vi "SlicePlane.vi"(0 "Plane dimensions (cm)":cluster{"x":dbl, "y":dbl, "z":dbl}={"x"=0.2, "y"=0.0, "z"=0.2} {"x" format="%.2f"; "z" format="%.2f"; "y" format="%.2f"}, 1 "strip (cm)":cluster{"radius":dbl, "h":dbl, "a":dbl}={"radius"=9.0, "h"=2.0, "a"=4.0} {"radius" format="%.2f"; "a" format="%.4f"; "h" format="%.4f"}, 2 "Plane":u16(ring)=2 items=["X-Y", "Z-Y", "X-Z"], 3 "freq (MHz)":dbl=4.7 format="%.2f", 4 "Geometry":u16(ring)=1 items=["single wedge", "dual wedge", "Outer Rec Hole", "Inner Rect Hole", "single strip", "dual strips", "Cap w/ Rect Cut", "middle pair", "middle w/ circ hole"], 6 "Points \t1":i32=10, 7 "Variables":T1={"sound spd (cm/s)"=150000, "time step (s)"=1e-09} {"time step (s)" format="%.2e"}, 8 "Points 2":i32=10, 14 "3D Surface":refnum<k7>(container)) -> (19 "raw data":dbl[][](array[numeric]) format="%.2f")   [LabVIEW 2022 SP3]
uses:
  <vilib>/Analysis/2dsp.llb/1D Convolution (DBL).vi
  <vilib>/Utility/file.llb/Write To Spreadsheet File (DBL).vi
  <vilib>/Platform/NI_3dgraph.lvlib
  <vilib>/Analysis/NI_AALBase.lvlib
  <vilib>/Analysis/NI_AALPro.lvlib
panel:
  in  "Case Constant\n(See Context Help)":bool
  in  "Boolean":bool
  out "data with axis":dbl[][](array[numeric]) format="%.4f"
  in  "save image":bool
  out "axial width (cm)":dbl format="%.4f"
  in  "lower h of strip or outer a":dbl format="%.2f"
  in  "Save Sheet":bool
  out "axial peak (cm)":dbl format="%.2f"
  out "3 dB beamwidth (cm)":dbl format="%.4f"
  out "lateral pressure (y or y or z)":cluster{"output":dbl[], "output":dbl[]}(graph)
  out "axial pressure (x or z or x)":cluster{dbl[], "output":dbl[]}(graph)
  # "y\ny\nz"
  # "x\nz\nx"
  # "For X-Y Pts 1 is for X and Pts 2 is for Y etc."
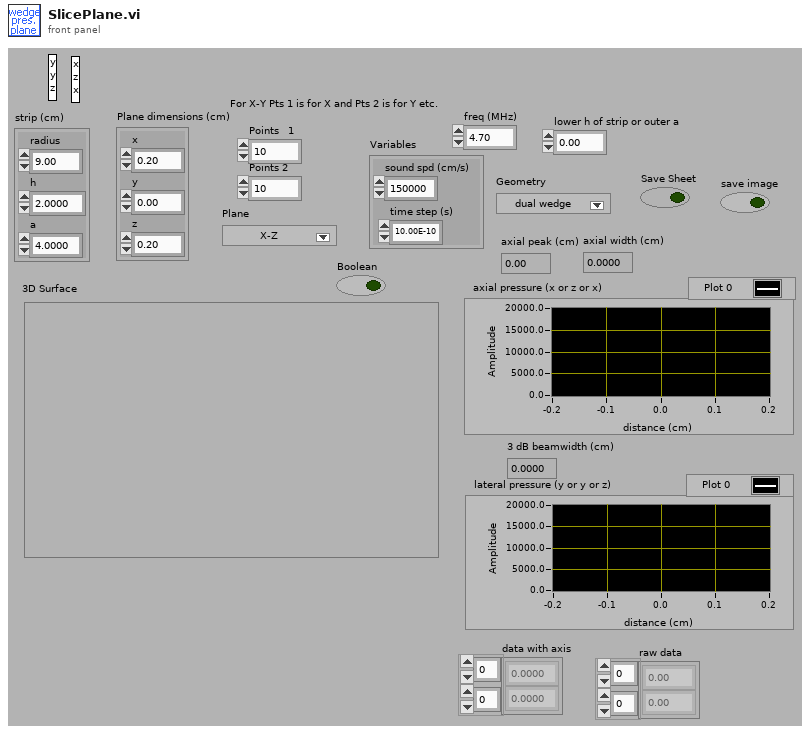
[diagram p1: front panel]
types:
  T1 = cluster{"sound spd (cm/s)":i32, "time step (s)":sgl}
  T2 = cluster{"Number of rings":i32, "sound spd (cm/s)":i32, "z span (cm)":dbl, "z steps":i32, "y span (cm)":dbl, "y steps":i32, "time step (s)":sgl, "z":dbl, "y":dbl, "ref delay":dbl, "freq (MHz)":dbl, "cycles":i32}
  T3 = cluster{"fixed plane":dbl, "fixed plane":dbl, "fixed plane":dbl}
  T4 = cluster{"axial pressure (z)":cluster{dbl[], "output":dbl[]}, "3 dB beamwidth (cm)":dbl, "lateral pressure (y)":cluster{"output":dbl[], "output":dbl[]}, "3 dB beamwidth (cm)":dbl}
  T5 = enum32{"existing file", "new file", "new or existing file", "existing dir", "new dir", "new or existing dir", "existing file (use LLBs)", "new file (use LLBs)", "new or existing file (use LLBs)", "new or existing file or directory (use LLBs)"}
  T6 = typedef "LVRectTypeDef.ctl" = cluster{"left":i16, "top":i16, "right":i16, "bottom":i16}
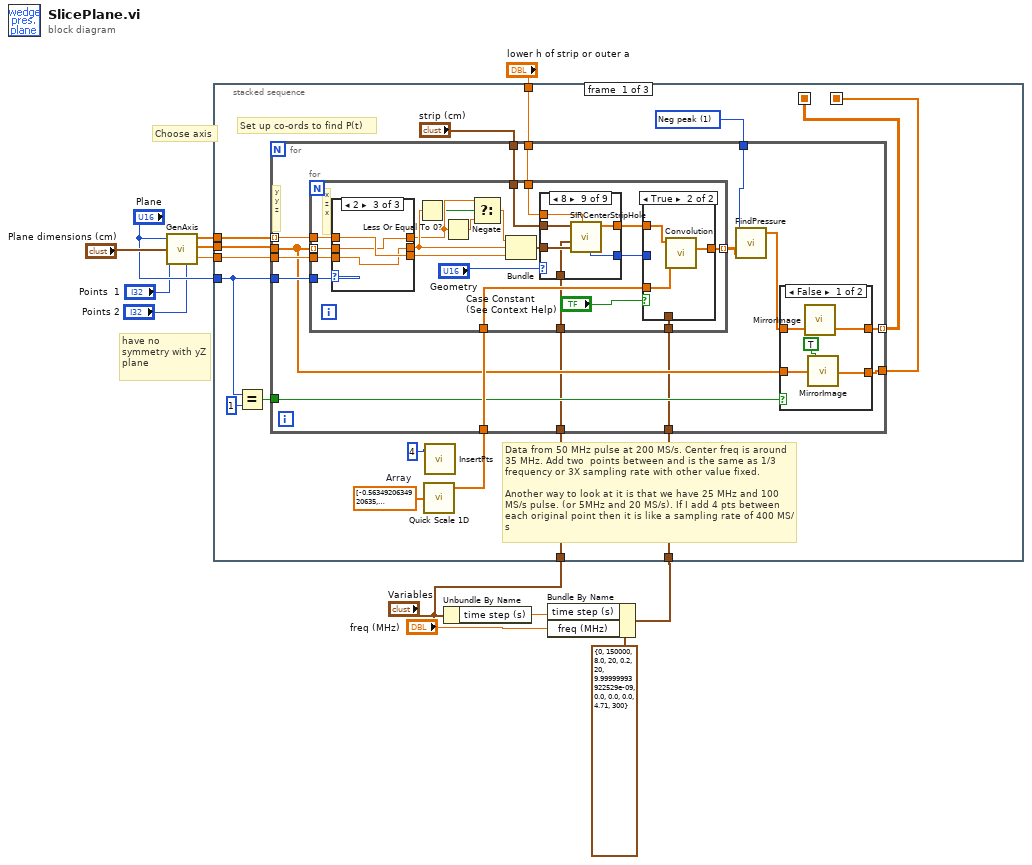
[diagram p0: block diagram]
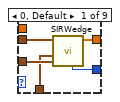
[diagram p3: hidden frame]
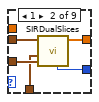
[diagram p4: hidden frame]
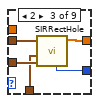
[diagram p5: hidden frame]
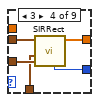
[diagram p6: hidden frame]
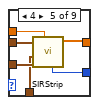
[diagram p7: hidden frame]
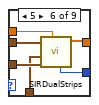
[diagram p8: hidden frame]
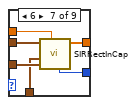
[diagram p9: hidden frame]
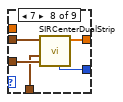
[diagram p10: hidden frame]
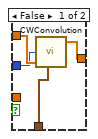
[diagram p11: hidden frame]
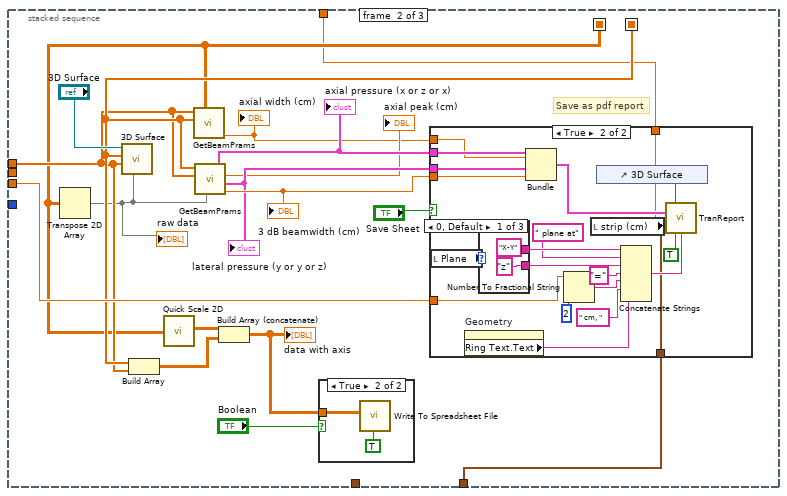
[diagram p14: hidden frame]
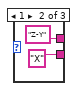
[diagram p17: hidden frame]
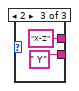
[diagram p18: hidden frame]
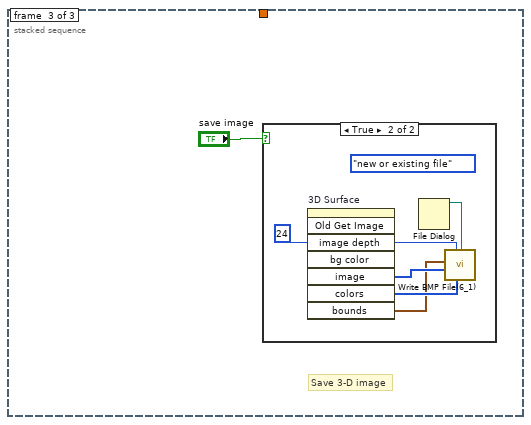
[diagram p19: hidden frame]
diagram:
  # "have no symmetry with yZ plane"
  # "Choose axis"
  n1 = call "GenAxis.vi"("Points2"="Points 2", "Plane"="Plane", "Plane dimensions (cm)"="Plane dimensions (cm)", "Points1"="Points \t1") -> ("outer index"=w5:dbl[], "inner index"=w11:dbl[], "fixed plane"=w6:dbl)  [unwired: 1 in]
  n2 = Unbundle By Name("Variables") -> ("time step (s)"=w8:sgl)
  n3 = Bundle By Name(cluster=T2 {"Number of rings"=0, "sound spd (cm/s)"=150000, "z span (cm)"=8.0, "z steps"=20, "y span (cm)"=0.2, "y steps"=20, "time step (s)"=1e-08, "z"=0.0, "y"=0.0, "ref delay"=0.0, "freq (MHz)"=4.71, "cycles"=300} ("Variables"), "time step (s)"=w8, "freq (MHz)"="freq (MHz)") -> (w4:T2)
  n4 = stacked-sequence {
    seq-local: [w21 _ _] -> [_ w144 _]
    seq-local: [w22 _ _] -> [_ w147 _]
    tunnel: "Plane" -> [w16 _ _]
    tunnel: w11 -> [w27 _ _]
    tunnel: w6 -> [w25 w149 _]
    tunnel: w5 -> [w23 w146 _]
    tunnel: w4 -> [w20 w138 _]
    tunnel: "Variables" -> [w15 _ _]
    tunnel: "lower h of strip or outer a" -> [w14 w140 _]
    frame #0 {
      w19 = u16 1 items=["Pos Peak", "Neg peak", "Steady State"] ("Pressure Calc")
      w26 = dbl[] [-0.5634920634920635, -0.6825396825396826, -0.8015873015873016, -0.9920634920634921, -1.1507936507936507, -1.3888888888888888, -1.992063492063492, -4.2063492063492065, -5.888888888888889, 13.023809523809524, 61.32539682539682, 92.83333333333333, 75.10317460317461, 18.126984126984127, -54.93650793650794, -109.60317460317461, -104.22222222222223, 18.134920634920636, 83.33333333333333, 27.27777777777778, -42.19047619047619, -45.63492063492063, 10.15079365079365, 49.05555555555556, 28.19047619047619, -5.658730158730159, -15.261904761904763, -4.4603174603174605, 7.984126984126984, 10.682539682539682, 5.809523809523809, -0.03968253968253968, -2.515873015873016, -1.4841269841269842, 1.0396825396825398, 2.0555555555555554, 0.9523809523809523, -0.6031746031746031, -1.007936507936508, -0.3968253968253968, 0.14285714285714285]  # Array
      # "Set up co-ords to find P(t)"
      # "Data from 50 MHz pulse at 200 MS/s. Center freq is around 35 MHz. Add two  points between and is the same as 1/3 frequency or 3X sampling rate with other value fixed.\n\nAnother way to look at it is that we have 25 MHz and 100 MS/s pulse. (or 5MHz and 20 MS/s). If I add 4 pts between each original point then it is like a sampling rate of 400 MS/s"
      n5 = Equal?(x=w16, y=1) -> (x = y?=w28:bool)
      n6 = call <vilib>:"Quick Scale 1D.vi"("X"=w26) -> ("Y[i]=X[i]/Max|X|"=w24:dbl[])  [unwired: 2 out]
      n7 = for {
        tunnel: w23 -> [w44] mode=indexing
        tunnel: "strip (cm)" -> [w43]
        tunnel: w24 -> [w42]
        tunnel: w16 -> [w41]
        tunnel: [w39] -> w21 mode=indexing
        tunnel: w19 -> [w40]
        tunnel: w28 -> [w37]
        tunnel: w27 -> [w34]
        tunnel: w25 -> [w36]
        tunnel: [w33] -> w22
        tunnel: w14 -> [w32]
        tunnel: w20 -> [w31]
        tunnel: w15 -> [w30]
        # "y\ny\nz"
        n8 = for {
          tunnel: w44 -> [w72]
          tunnel: w43 -> [w65]
          tunnel: w42 -> [w69]
          tunnel: w41 -> [w70]
          tunnel: [w67] -> w38 mode=indexing
          tunnel: w34 -> [w64] mode=indexing
          tunnel: w36 -> [w63]
          tunnel: w32 -> [w54]
          tunnel: w31 -> [w53]
          tunnel: w30 -> [w52]
          # "x\nz\nx"
          n9 = case shown="2" w70 {
            tunnel: [w130 w132 w136] -> w60
            tunnel: w72 -> [w131 w134 w137]
            tunnel: [w129 w133 w137] -> w71
            tunnel: [w131 w134 w135] -> w62
            tunnel: w64 -> [w130 w133 w136]
            tunnel: w63 -> [w129 w132 w135]
            frame 0, Default {
            }
            frame 1 {
            }
            frame 2 {
            }
          }
          n10 = Less Or Equal To 0?(x=w62) -> (x <= 0?=w58:bool)
          n11 = Negate(x=w60) -> (-x=w61:dbl)
          n12 = Select(t=w60, s=w58, f=w61) -> (s? t:f=w59:dbl)
          n13 = Bundle("fixed plane"=w59, "fixed plane"=w62, "fixed plane"=w71) -> (w66:T3)  [unwired: 1 in]
          n14 = case shown="8" "Geometry" {
            tunnel: [w77 w80 w87 w89 w93 w102 w108 w113 w119] -> w68
            tunnel: w66 -> [w76 w81 w85 w91 w98 w104 w109 w114 w120]
            tunnel: w65 -> [w75 w82 w86 w92 w96 w103 w110 w115 w121]
            tunnel: [w74 w79 w84 w90 w97 w101 w107 w112 w118] -> w57
            tunnel: w54 -> [_ _ _ _ w95 w99 w106 _ w116]
            tunnel: w52 -> [w73 w78 w83 w88 w94 w100 w105 w111 w117]
            frame 0, Default {
              n15 = call "SIRWedge.vi"("P"=w76, "Variables"=w73, "strip"=w75) -> ("h wedge"=w77:dbl[], "wedge delay"=w74:i32)  [unwired: 1 in, 6 out]
            }
            frame 1 {
              n16 = call "SIRDualSlices.vi"("P"=w81, "Variables"=w78, "strip"=w82) -> ("h outer strips"=w80:dbl[], "delay out"=w79:i32)  [unwired: 2 in, 5 out]
            }
            frame 2 {
              n17 = call "SIRRectHole.vi"("P"=w85, "Variables"=w83, "strip"=w86) -> ("h rect"=w87:dbl[], "delay out"=w84:i32)  [unwired: 3 in, 4 out]
            }
            frame 3 {
              n18 = call "SIRRect.vi"("P"=w91, "Variables"=w88, "strip"=w92) -> ("h rect"=w89:dbl[], "delay out"=w90:i32)  [unwired: 5 in, 2 out]
            }
            frame 4 {
              n19 = call "SIRStrip.vi"("lower h of strip"=w95, "P"=w98, "Variables"=w94, "strip"=w96) -> ("h out"=w93:dbl[], "delay out"=w97:i32)  [unwired: 4 in, 2 out]
            }
            frame 5 {
              n20 = call "SIRDualStrips.vi"("lower h of strip"=w99, "P"=w104, "Variables"=w100, "strip"=w103) -> ("h out"=w102:dbl[], "delay out"=w101:i32)  [unwired: 4 in, 2 out]
            }
            frame 6 {
              n21 = call "SIRRectInCap.vi"("outer a"=w106, "P"=w109, "Variables"=w105, "strip"=w110) -> ("h rect"=w108:dbl[], "delay out"=w107:i32)  [unwired: 4 in, 2 out]
            }
            frame 7 {
              n22 = call "SIRCenterDualStrip.vi"("P"=w114, "Variables"=w111, "strip"=w115) -> ("h out"=w113:dbl[], "delay out"=w112:i32)  [unwired: 5 in, 2 out]
            }
            frame 8 {
              n23 = call "SIRCenterStripHole.vi"("center hole"=w116, "P"=w120, "Variables"=w117, "strip"=w121) -> ("h out"=w119:dbl[], "delay out"=w118:i32)  [unwired: 4 in, 2 out]
            }
          }
          n24 = case shown="True" "Case Constant\n(See Context Help)" {
            tunnel: w69 -> [_ w128]
            tunnel: w68 -> [w125 w126]
            tunnel: [w123 w127] -> w67
            tunnel: w57 -> [w124 _]
            tunnel: w53 -> [w122 _]
            frame False {
              n25 = call "CWConvolution.vi"("delay pts"=w124, "h(r,t)"=w125, "Variables"=w122) -> ("X*Y"=w123:dbl[])  [unwired: 3 in, 1 out]
            }
            frame True {
              n26 = call-poly <vilib>:"Convolution.vi"("Y"=w128, "X"=w126) -> ("X * Y"=w127:dbl[])  [unwired: 8 in, 1 out]
            }
          }
        }
        n27 = call "FindPressure.vi"("Pressure Calc"=w40, "Input"=w38) -> ("Pressures"=w35:dbl[])  [unwired: 5 in]
        n28 = case shown="False" w37 {
          tunnel: [w49 w51] -> w39
          tunnel: w35 -> [w48 w51]
          tunnel: w34 -> [w46 w50]
          tunnel: [w45 w50] -> w33
          frame False {
            n29 = call "MirrorImage.vi"("input"=w48) -> ("output"=w49:dbl[])  [unwired: 2 in]
            n30 = call "MirrorImage.vi"("input"=w46, "neg?"=TRUE) -> ("output"=w45:dbl[])  [unwired: 1 in]
          }
          frame True {
          }
        }
      }
      n31 = call "InsertPts.vi"("pts to insert"=4) -> ()  [unwired: 1 in, 1 out]
    }
    frame #1 {
      # "Save as pdf report"
      n32 = Transpose 2D Array(2D array=w144) -> (transposed array=w145:dbl[][])
      "raw data" <- w145
      n33 = call <vilib>:"3D Surface.vi"("z matrix"=w145, "y vector"=w146, "x vector"=w147, "3D graph"="3D Surface") -> ()  [unwired: 6 in, 2 out]
      n34 = Build Array(w147, w146) -> (w148:dbl[][])
      n35 = call <vilib>:"Quick Scale 2D.vi"("X"=w144) -> ("Yij=Xij/Max|X|"=w143:dbl[][])  [unwired: 2 out]
      n36 = call "GetBeamPrams.vi"("data"=w144, "ycoords"=w147, "x coords"=w146) -> ("3 dB beamwidth (cm)"=w139:dbl)  [unwired: 2 in, 3 out]
      "axial width (cm)" <- w139
      n37 = call "GetBeamPrams.vi"("data"=w145, "ycoords"=w146, "x coords"=w147) -> ("3 dB beamwidth (cm)"=w154:dbl, "lateral pressure (y)"=w153:cluster{"output":dbl[], "output":dbl[]}, "axial peak (cm)"=→"axial peak (cm)":dbl, "axial pressure (z)"=w155:cluster{dbl[], "output":dbl[]})  [unwired: 2 in]
      "3 dB beamwidth (cm)" <- w154
      "lateral pressure (y or y or z)" <- w153
      "axial pressure (x or z or x)" <- w155
      n38 = Build Array (concatenate)(w143, w148) -> (w142:dbl[][])
      "data with axis" <- w142
      n39 = case shown="True" "Boolean" {
        tunnel: w142 -> [_ w157]
        frame False {
        }
        frame True {
          n40 = call-poly <vilib>:"Write To Spreadsheet File.vi"("transpose? (no:F)"=TRUE, "2D data"=w157) -> ()  [unwired: 6 in, 1 out]
        }
      }
      n41 = case shown="True" "Save Sheet" {
        tunnel: w155 -> [_ w176]
        tunnel: w153 -> [_ w175]
        tunnel: w154 -> [_ w174]
        tunnel: w149 -> [_ w166]
        tunnel: w140 -> [_ w161]
        tunnel: w139 -> [_ w159]
        tunnel: w138 -> [_ w158]
        frame False {
        }
        frame True {
          n42 = local read "Plane"() -> (w171:u16)
          n43 = property on="Geometry" class="Ring (strict)"() -> ("Ring Text.Text"=w160:string)  [unwired: 2 in, 2 out]
          n44 = case shown="0, Default" w171 {
            tunnel: ["X-Y" "Z-Y" "X-Z"] -> w170
            tunnel: ["z" "X" " Y"] -> w167
            frame 0, Default {
            }
            frame 1 {
            }
            frame 2 {
            }
          }
          n45 = Bundle("axial pressure (z)"=w176, "3 dB beamwidth (cm)"=w159, "lateral pressure (y)"=w175, "3 dB beamwidth (cm)"=w174) -> (w173:T4)  [unwired: 1 in]
          n46 = Number To Fractional String(number=w166, precision (6)=2) -> (F-format string=w165:string)  [unwired: 2 in]
          n47 = local read "strip (cm)"() -> (w178:cluster{"radius":dbl, "h":dbl, "a":dbl})
          n48 = control-ref of="3D Surface"() -> (w177:refnum<vi>)
          n49 = Concatenate Strings(w170, " plane at", w167, "=", w165, " cm, ", w160) -> (w164:string)
          n50 = call "TranReport.vi"("3D Surface"=w177, "Output Cluster"=w173, "Trans Geometry"=w178, "Center Hole"=w161, "Variables"=w158, "case"=TRUE, "ring locations"=w164) -> ()  [unwired: 9 in]
        }
      }
    }
    frame #2 {
      # "Save 3-D image"
      n51 = case shown="True" "save image" {
        frame False {
        }
        frame True {
          (unwired) T5."new or existing file" ("select mode (2)")
          w190 = 24
          n52 = invoke on="3D Surface" class="AXCont" method="Old Get Image"("image depth"=w190) -> ("image"=w188:u8[], "colors"=w189:u32[], "bounds"=w187:T6)  [unwired: 7 in, 5 out]
          n53 = File Dialog() -> (3:w186:path)  [unwired: 7 in, 3 out]
          n54 = call <vilib>:"Write BMP File(6_1).vi"("color table"=w189, "depth"=w190, "flattened image data"=w188, "rect"=w187, "path to BMP file"=w186) -> ()  [unwired: 5 in, 2 out]
        }
      }
    }
  }
